vi "Set message.vi"(10 "WampMessage MsgPack":refnum<class "WampMessage MsgPack.lvclass">, 11 "InvocationHandler MsgPack in":refnum<class "InvocationHandler MsgPack.lvclass">) -> (3 "InvocationHandler MsgPack out":refnum<class "InvocationHandler MsgPack.lvclass">)   [LabVIEW 2020, in "wamplv.lvlib" / "InvocationHandler MsgPack.lvclass"]
uses:
  InvocationHandler MsgPack.lvclass
  InvocationHandler MsgPack.lvclass/InvocationHandler MsgPack.ctl
  SerialisedMessages/MsgPackMessage/WampMessage MsgPack.lvclass
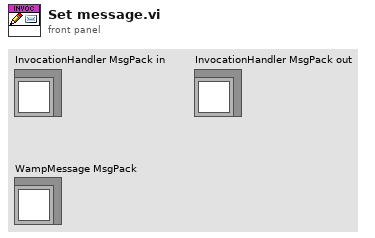
[diagram p1: front panel]
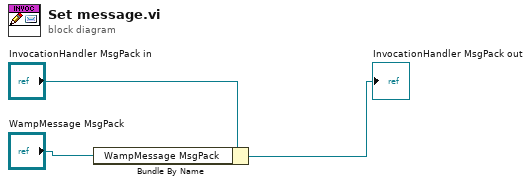
[diagram p0: block diagram]
diagram:
  n1 = Bundle By Name(cluster="InvocationHandler MsgPack in", "WampMessage MsgPack"="WampMessage MsgPack") -> (→"InvocationHandler MsgPack out":refnum<class "InvocationHandler MsgPack.lvclass">)
